vi "RfSwitch_GUI.vi"(0 "VISA_IN":refnum<visa-resource-name>="GPIB0::29::INSTR", 11 "error in":errorcluster, 12 "Source":enum16{"RFSM", "PNA"}(ring), 14 "T/R":enum16{"TX", "RX"}(ring)) -> (2 "SwitchViRef":refnum<vi>, 4 "visa_out":refnum<visa-resource-name>, 15 "error out":errorcluster)   [LabVIEW 2018]
panel:
  in  "stop":bool
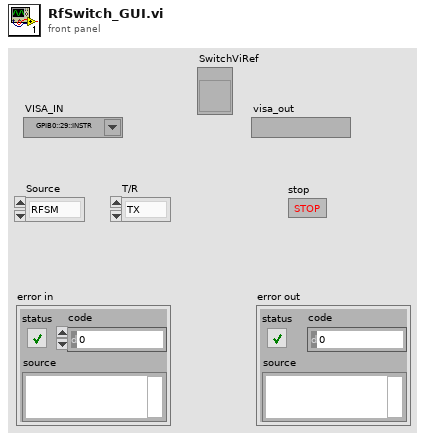
[diagram p1: front panel]
types:
  T1 = enum32{"Invalid", "Standard", "Closed", "Hidden", "Minimized", "Maximized"}
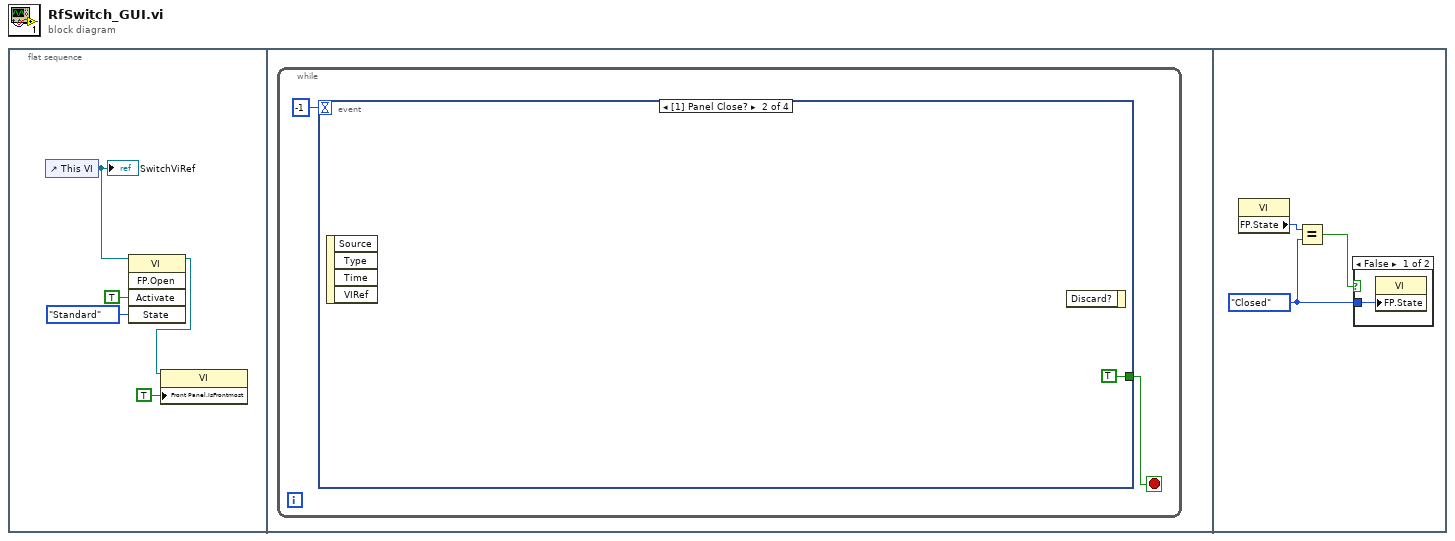
[diagram p0: block diagram]
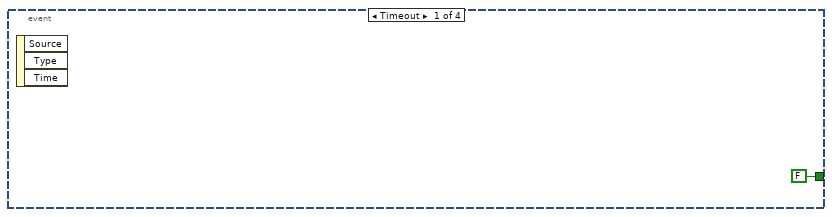
[diagram p2: hidden frame]
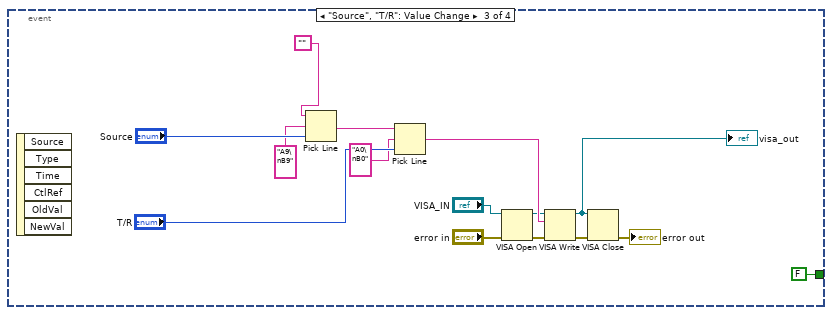
[diagram p3: hidden frame]
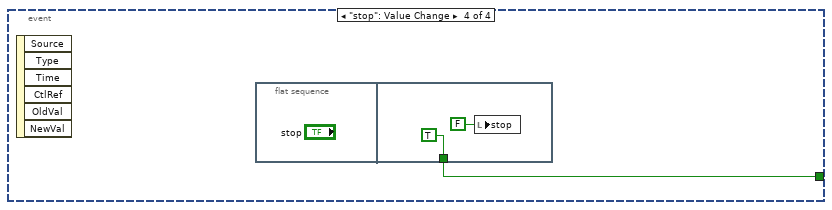
[diagram p4: hidden frame]
diagram:
  n1 = flat-sequence {
    frame #0 {
      n2 = control-ref of="This VI"() -> (w5:refnum<vi>)
      "SwitchViRef" <- w5
      n3 = invoke class="VI" method="FP.Open"(reference=w5, "Activate"=TRUE ("Activate?"), "State"=T1."Standard") -> (reference out=w2:refnum<vi>)  [unwired: 2 in, 4 out]
      n4 = property class="VI"(reference=w2, "Front Panel.IsFrontmost"=TRUE ("Front Panel Window:Is Frontmost")) -> ()  [unwired: 1 in, 2 out]
    }
    frame #1 {
      n5 = while {
        stop <- w6 stop-if-true
        n6 = event shown="[1] Panel Close?" {
          selector: _ -> [_ _ _ _]
          dyn-events: _ -> [_ _ _ _]
          timeout: -1 -> [_ _ _ _]
          tunnel: [FALSE TRUE FALSE w25] -> w6
          event Timeout {
            n7 = event-data() -> ()  [unwired: 1 in, 3 out]
          }
          event Panel Close? {
            n8 = event-data() -> ()  [unwired: 1 in, 4 out]
            n9 = event-data() -> ()  [unwired: 2 in, 1 out]
          }
          event "Source", "T/R": Value Change {
            n10 = event-data() -> ()  [unwired: 1 in, 6 out]
            n11 = Pick Line(string ("")="", multi-line string="A9\nB9", line index="Source") -> (output string=w22:string)
            n12 = Pick Line(string ("")=w22, multi-line string="A0\nB0", line index="T/R") -> (output string=w23:string)
            n13 = VISA Open(error in (no error)="error in", VISA resource name="VISA_IN") -> (VISA resource name=w15:refnum<visa-resource-name>, error out=w16:errorcluster)  [unwired: 3 in]
            n14 = VISA Write(VISA resource name=w15, write buffer=w23, error in (no error)=w16) -> (VISA resource name out=w17:refnum<visa-resource-name>, error out=w14:errorcluster)  [unwired: 1 out]
            "visa_out" <- w17
            n15 = VISA Close(VISA resource name=w17, error in (no error)=w14) -> (error out=→"error out":errorcluster)
          }
          event "stop": Value Change {
            n16 = event-data() -> ()  [unwired: 1 in, 6 out]
            n17 = flat-sequence {
              tunnel: [TRUE] -> w25
              frame #0 {
              }
              frame #1 {
                n18 = local write "stop"(FALSE ("stop")) -> ()
              }
            }
          }
        }
      }
    }
    frame #2 {
      w29 = T1."Closed" ("Front Panel Window:State")
      n19 = property class="VI"() -> ("FP.State"=w30:T1)  [unwired: 2 in, 2 out]
      n20 = Equal?(x=w30, y=w29) -> (x = y?=w28:bool)
      n21 = case shown="False" w28 {
        tunnel: w29 -> [w31 _]
        frame False {
          n22 = property class="VI"("FP.State"=w31) -> ()  [unwired: 2 in, 2 out]
        }
        frame True {
        }
      }
    }
  }
